vi "Sweep.vi"(8 "error in (no error)":errorcluster, 11 "Spectrum Recorder in":refnum<class "Spectrum Recorder too.lvclass">) -> (0 "error out":errorcluster, 3 "Spectrum Recorder out":refnum<class "Spectrum Recorder too.lvclass">)   [LabVIEW 2016, in "Spectrum Recorder too.lvclass"]
uses:
  Spectrum Recorder too.lvclass
  C:/github/Measure_core/Worker/Worker.lvclass
  Measure_core/Worker/Worker.lvclass/Worker.ctl
  Spectrum Recorder too.lvclass/Spectrum Recorder too.ctl
  Measure_core/Template Module/Read Active.vi
  NHMFL_Core/Libraries/Red Pitaya/RP Core/RP Transceiver/RP Transceiver.lvclass
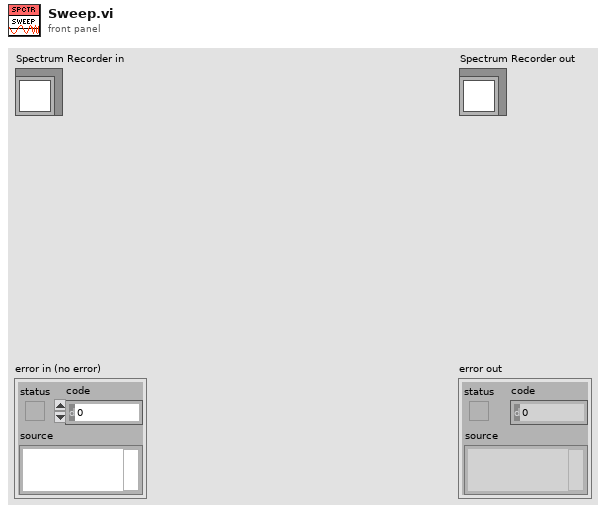
[diagram p1: front panel]
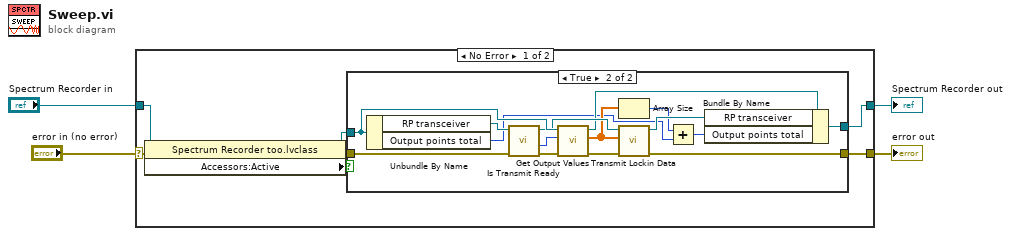
[diagram p0: block diagram]
diagram:
  n1 = case shown="No Error" "error in (no error)" {
    selector: "error in (no error)" -> [w10 w30]
    tunnel: [w9 w30] -> w3
    tunnel: [w11 w29] -> w1
    tunnel: "Spectrum Recorder in" -> [w7 w29]
    frame No Error {
      n2 = property class="Spectrum Recorder too.lvclass"(reference=w7, error in=w10) -> (reference out=w6:refnum<class "Spectrum Recorder too.lvclass">, error out=w8:errorcluster, "Accessors:Active"=w5:bool)
      n3 = case shown="True" w5 {
        tunnel: w6 -> [w13 w26]
        tunnel: w8 -> [w12 w27]
        tunnel: [w13 w19] -> w11
        tunnel: [w12 w18] -> w9
        frame False {
        }
        frame True {
          n4 = Unbundle By Name(w26) -> ("RP transceiver"=w28:refnum<class "RP Transceiver.lvclass">, "Output points total"=w15:i64)
          n5 = call-dynamic "Is Transmit Ready.vi"("error in (no error)"=w27, "RP Instrument in"=w28) -> ("error out"=w24:errorcluster, "Unused buffer"=w25:i32, "RP Instrument out"=w23:refnum<class "RP Transceiver.lvclass">)  [unwired: 6 in, 1 out]
          n6 = call-dynamic "Get Output Values.vi"("error in (no error)"=w24, "Number of points"=w25, "Spectrum Recorder in"=w26) -> ("error out"=w22:errorcluster, "Output values"=w17:dbl[], "Spectrum Recorder out"=w21:refnum<class "Spectrum Recorder too.lvclass">)  [unwired: 6 in]
          n7 = Array Size(array=w17) -> (size(s)=w16:i32)
          n8 = call-dynamic "Transmit Lockin Data.vi"("error in (no error)"=w22, "Data"=w17, "RP Transceiver in"=w23) -> ("error out"=w18:errorcluster, "RP Transceiver out"=w20:refnum<class "RP Transceiver.lvclass">)  [unwired: 6 in, 1 out]
          n9 = Add(x=w16, y=w15) -> (x+y=w14:i64)
          n10 = Bundle By Name(cluster=w21, "RP transceiver"=w20, "Output points total"=w14) -> (w19:refnum<class "Spectrum Recorder too.lvclass">)
        }
      }
    }
    frame Error {
    }
  }
  "error out" <- w3
  "Spectrum Recorder out" <- w1
